vi "PH_StatusHandler.PC set Status.vi"(0 "i ref in":refnum<vi>, 3 "Status":T1 items=["no info", "off/false/out", "on/true/in", "Failure", "Alarm", "Status 1", "Status 2", "Status 3"], 4 "Blinking (false)":bool, 5 "error in (no error)":errorcluster, 7 "Tip Strip":string="N/A") -> (14 "i ref out":refnum<vi>, 19 "error out":errorcluster)   [LabVIEW 2014, in "PH_StatusHandler.lvlib"]
doc: "This VI sets the connected GUI element and updates the DIM service."
uses:
  PH_StatusHandler.lvlib
  PH_StatusHandler.Status.ctl
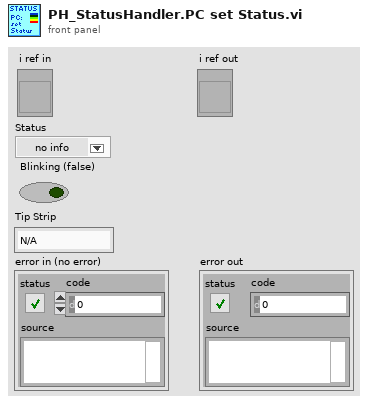
[diagram p1: front panel]
types:
  T1 = typedef "PH_StatusHandler.lvlib/PH_StatusHandler.Status.ctl" = i16
  T2 = typedef "PH_StatusHandler.lvlib/PH_StatusHandler.i attribute.ctl" = cluster{"GUI Ref":refnum<vi>, "Value":T1, "Service ID":i32}
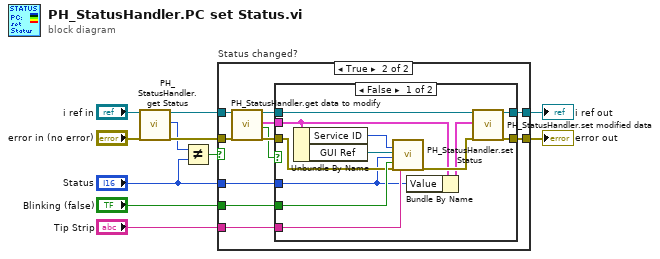
[diagram p0: block diagram]
diagram:
  n1 = call "PH_StatusHandler.get Status.vi"("VI in"="i ref in", "error in"="error in (no error)") -> ("VI out"=w4:refnum<vi>, "Status"=w3:T1, "error out"=w6:errorcluster)  [unwired: 15 in]
  n2 = Not Equal?(x=w3, y="Status") -> (x != y?=w1:bool)
  n3 = case "Status changed?" shown="True" w1 {
    tunnel: "Blinking (false)" -> [_ w24]
    tunnel: "Tip Strip" -> [_ w23]
    tunnel: [w12 w22] -> w8
    tunnel: [w13 w18] -> w7
    tunnel: w6 -> [w12 w16]
    tunnel: w4 -> [w13 w15]
    tunnel: "Status" -> [_ w14]
    frame False {
    }
    frame True {
      n4 = call "PH_StatusHandler.get data to modify.vi"("i ref in"=w15, "error in (no error)"=w16) -> ("i ref out"=w20:refnum<vi>, "i attribute"=w19:T2, "timed out"=w17:bool, "error out"=w21:errorcluster)  [unwired: 14 in]
      n5 = case shown="False" w17 {
        tunnel: w24 -> [w36 _]
        tunnel: w23 -> [w35 _]
        tunnel: [w34 w37] -> w22
        tunnel: w21 -> [w33 w37]
        tunnel: w20 -> [w32 w38]
        tunnel: w19 -> [w28 _]
        tunnel: w14 -> [w26 _]
        tunnel: [w25 w38] -> w18
        frame False {
          n6 = Unbundle By Name(w28) -> ("Service ID"=w30:i32, "GUI Ref"=w31:refnum<vi>)
          n7 = call "PH_StatusHandler.set Status.vi"("Service ID Status"=w30, "Ring in"=w31, "Status"=w26, "Blinking (false)"=w36, "error in (no error)"=w33, "Tip Strip"=w35) -> ("error out"=w29:errorcluster)  [unwired: 13 in]
          n8 = Bundle By Name(cluster=w28, "Value"=w26) -> (w27:T2)
          n9 = call "PH_StatusHandler.set modified data.vi"("i ref in"=w32, "i attribute"=w27, "error in (no error)"=w29) -> ("i ref out"=w25:refnum<vi>, "error out"=w34:errorcluster)  [unwired: 15 in]
        }
        frame True {
        }
      }
    }
  }
  "error out" <- w8
  "i ref out" <- w7
